vi "Post-Build Custom Action.vi"(10 "Variant":variant) -> (0 "error out":errorcluster)   [LabVIEW 2015, in "HTML Help File Tools.lvlib"]
uses:
  HTML Help File Tools.lvlib
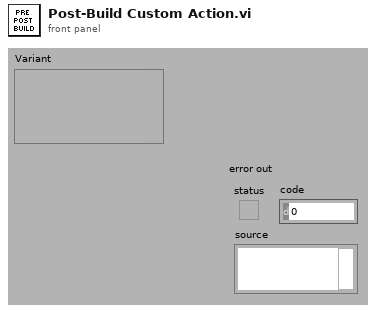
[diagram p1: front panel]
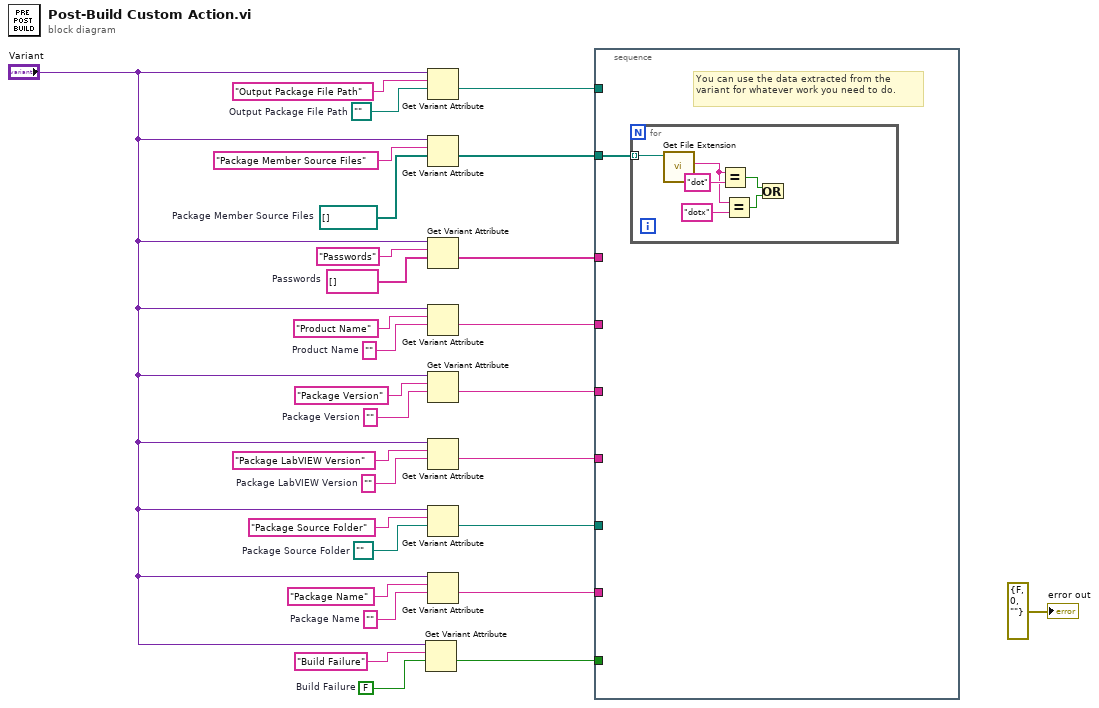
[diagram p0: block diagram]
diagram:
  w3 = FALSE  # Build Failure
  w13 = path ""  # Package Source Folder
  w14 = ""  # Package Name
  w17 = ""  # Package LabVIEW Version
  w19 = ""  # Package Version
  w21 = ""  # Product Name
  w24 = string[] []  # Passwords
  w26 = path[] []  # Package Member Source Files
  w28 = path ""  # Output Package File Path
  n1 = Get Variant Attribute(Variant="Variant", name="Build Failure", default value (empty Variant)=w3) -> (value=w1:bool)  [unwired: 1 in, 3 out]
  n2 = Get Variant Attribute(Variant="Variant", name="Output Package File Path", default value (empty Variant)=w28) -> (value=w12:path)  [unwired: 1 in, 3 out]
  n3 = Get Variant Attribute(Variant="Variant", name="Package Member Source Files", default value (empty Variant)=w26) -> (value=w11:path[])  [unwired: 1 in, 3 out]
  n4 = Get Variant Attribute(Variant="Variant", name="Passwords", default value (empty Variant)=w24) -> (value=w10:string[])  [unwired: 1 in, 3 out]
  n5 = Get Variant Attribute(Variant="Variant", name="Product Name", default value (empty Variant)=w21) -> (value=w9:string)  [unwired: 1 in, 3 out]
  n6 = Get Variant Attribute(Variant="Variant", name="Package Version", default value (empty Variant)=w19) -> (value=w8:string)  [unwired: 1 in, 3 out]
  n7 = Get Variant Attribute(Variant="Variant", name="Package LabVIEW Version", default value (empty Variant)=w17) -> (value=w7:string)  [unwired: 1 in, 3 out]
  n8 = Get Variant Attribute(Variant="Variant", name="Package Source Folder", default value (empty Variant)=w13) -> (value=w6:path)  [unwired: 1 in, 3 out]
  n9 = Get Variant Attribute(Variant="Variant", name="Package Name", default value (empty Variant)=w14) -> (value=w5:string)  [unwired: 1 in, 3 out]
  n10 = stacked-sequence {
    tunnel: w12 -> [_]
    tunnel: w11 -> [w30]
    tunnel: w10 -> [_]
    tunnel: w9 -> [_]
    tunnel: w8 -> [_]
    tunnel: w7 -> [_]
    tunnel: w6 -> [_]
    tunnel: w5 -> [_]
    tunnel: w1 -> [_]
    frame #0 {
      # "You can use the data extracted from the variant for whatever work you need to do."
      n11 = for {
        tunnel: w30 -> [w36] mode=indexing
        n12 = call <vilib>:"Get File Extension.vi"("file"=w36) -> ("lowercase file extension"=w34:string)  [unwired: 6 in, 4 out]
        n13 = Equal?(x=w34, y="dot") -> (x = y?=w32:bool)
        n14 = Equal?(x=w34, y="dotx") -> (x = y?=w31:bool)
        n15 = Or(x=w32, y=w31) -> ()  [unwired: 1 out]
      }
    }
  }
  "error out" <- errorcluster {"status"=FALSE, "code"=0, "source"=""} ("error out")
